vi "Event Is Nested.vi"(10 "Alias":string, 11 "Base Queue jettl in":refnum<class "Base Queue jettl.lvclass">) -> (2 "Event Is Nested?":bool)   [LabVIEW 2021, in "jettl.lvlib" / "Base Queue jettl.lvlib" / "Base Queue jettl.lvclass"]
uses:
  Base Queue jettl.lvclass
  Base Queue jettl.lvclass/Base Queue jettl.ctl
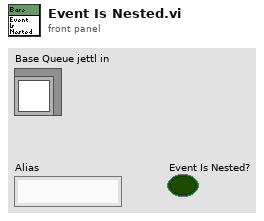
[diagram p1: front panel]
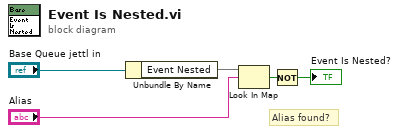
[diagram p0: block diagram]
diagram:
  # "Alias found?"
  n1 = Unbundle By Name("Base Queue jettl in") -> ("Event Nested"=w5:map{string, refnum<data-value>})
  n2 = Look In Map(map=w5, key="Alias") -> (key not found?=w4:bool)  [unwired: 1 in, 1 out]
  n3 = Not(x=w4) -> (.not. x?=→"Event Is Nested?":bool)
